vi "VA CoAP - Message - Option Insert - 11 Uri-Path.vi"(7 "URI-Path":string, 9 "Current Option Delta":u8, 10 "CoAP Message IN":string) -> (2 "New Option Delta":u8, 3 "CoAP Message OUT":string)   [LabVIEW 2020]
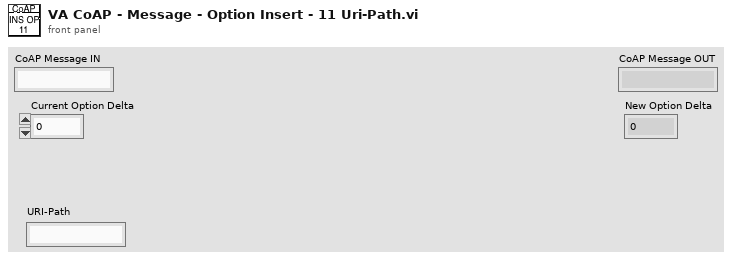
[diagram p1: front panel]
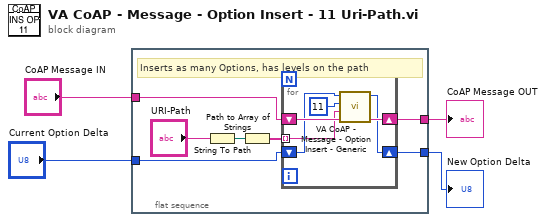
[diagram p0: block diagram]
diagram:
  n1 = flat-sequence {
    tunnel: "CoAP Message IN" -> [w11]
    tunnel: [w10] -> w3
    tunnel: "Current Option Delta" -> [w9]
    tunnel: [w8] -> w1
    frame #0 {
      # "Inserts as many Options, has levels on the path"
      n2 = String To Path(string="URI-Path") -> (path=w6:path)
      n3 = Path to Array of Strings(0:w6) -> (2:w5:string[])  [unwired: 1 out]
      n4 = for {
        shift-right: [w16] -> w10
        shift-left: w11 -> [w17]
        shift-right: [w14] -> w8
        shift-left: w9 -> [w15]
        tunnel: w5 -> [w12] mode=indexing
        n5 = call "VA CoAP - Message - Option Insert - Generic.vi"("CoAP Message IN"=w17, "New Message Element"=w12, "Current Delta on Evaluation"=u8 11 ("Current Option Delta"), "Current Option Delta in"=w15) -> ("CoAP Message OUT"=w16:string, "Current Option Delta out"=w14:u8)  [unwired: 6 in]
      }
    }
  }
  "CoAP Message OUT" <- w3
  "New Option Delta" <- w1
